vi "Configure DMM.vi"(5 "Resolution in Digits":T1(ring)=enum."5 1/2", 7 "Range":dbl=10.0 format="%.2f", 8 "error in (no error)":errorcluster, 9 "Measurement Type":T2(ring), 11 "niDMM in":refnum<class "niDMM.lvclass">) -> (0 "error out":errorcluster, 3 "niDMM out":refnum<class "niDMM.lvclass">)   [LabVIEW 2021, in "niDMM.lvclass"]
doc: "Configures the NI-DMM"
uses:
  niDMM.lvclass
  niDMM.lvclass/niDMM.ctl
  <instrlib>/niDMM/nidmm.llb/niDMM Resolution in Digits.ctl
  <instrlib>/niDMM/nidmm.llb/niDMM Configure Measurement Digits.vi
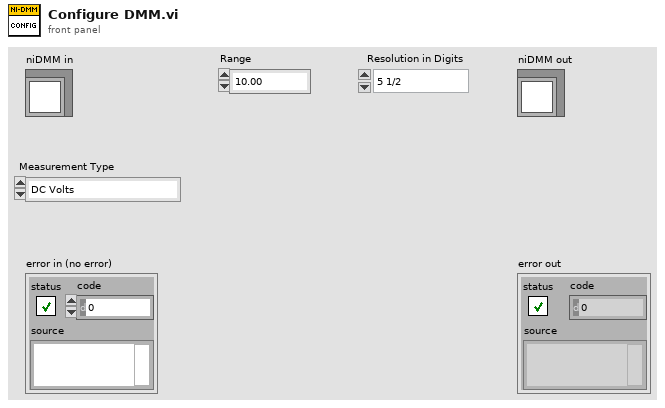
[diagram p1: front panel]
types:
  T1 = enum32{"3 1/2", "4 1/2", "5 1/2", "6 1/2", "7 1/2"}
  T2 = enum32{"DC Volts", "AC Volts", "DC Current", "AC Current", "2-wire Resistance", "4-wire Resistance", "Diode", "Frequency", "Period", "AC Volts DC Coupled", "Capacitance", "Inductance", "Temperature"}
  T3 = typedef "niDMM Resolution in Digits.ctl" = dbl
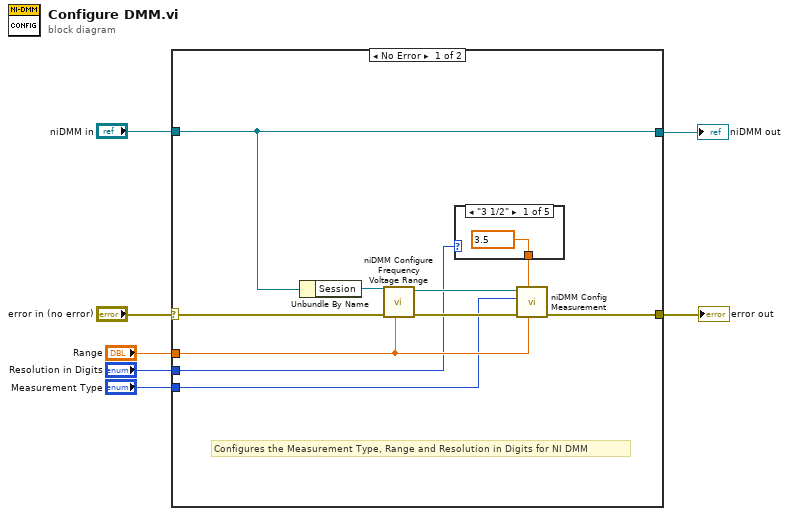
[diagram p0: block diagram]
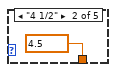
[diagram p2: hidden frame]
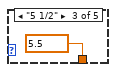
[diagram p3: hidden frame]
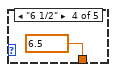
[diagram p4: hidden frame]
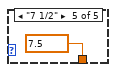
[diagram p5: hidden frame]
diagram:
  n1 = case shown="No Error" "error in (no error)" {
    selector: "error in (no error)" -> [w17 w23]
    tunnel: "niDMM in" -> [w16 w24]
    tunnel: [w16 w24] -> w5
    tunnel: [w15 w23] -> w4
    tunnel: "Range" -> [w10 _]
    tunnel: "Resolution in Digits" -> [w9 _]
    tunnel: "Measurement Type" -> [w8 _]
    frame No Error {
      # "Configures the Measurement Type, Range and Resolution in Digits for NI DMM"
      n2 = Unbundle By Name(w16) -> ("Session"=w11:refnum<k15>)
      n3 = call <instrlib>:"niDMM Configure Frequency Voltage Range.vi"("Frequency Voltage Range"=w10, "error in (no error)"=w17, "instrument handle"=w11) -> ("error out"=w14:errorcluster, "instrument handle out"=w13:refnum<k15>)  [unwired: 7 in]
      n4 = case shown="\"3 1/2\"" w9 {
        tunnel: [w18 w19 w20 w21 w22] -> w12
        frame "3 1/2" {
          w18 = T3 3.5 items=["3 1/2"=3.5, "4 1/2"=4.5, "5 1/2"=5.5, "6 1/2"=6.5, "7 1/2"=7.5] ("Resolution in Digits")
        }
        frame "4 1/2" {
          w19 = T3 4.5 items=["3 1/2"=3.5, "4 1/2"=4.5, "5 1/2"=5.5, "6 1/2"=6.5, "7 1/2"=7.5] ("Resolution in Digits")
        }
        frame "5 1/2" {
          w20 = T3 5.5 items=["3 1/2"=3.5, "4 1/2"=4.5, "5 1/2"=5.5, "6 1/2"=6.5, "7 1/2"=7.5] ("Resolution in Digits")
        }
        frame "6 1/2" {
          w21 = T3 6.5 items=["3 1/2"=3.5, "4 1/2"=4.5, "5 1/2"=5.5, "6 1/2"=6.5, "7 1/2"=7.5] ("Resolution in Digits")
        }
        frame "7 1/2" {
          w22 = T3 7.5 items=["3 1/2"=3.5, "4 1/2"=4.5, "5 1/2"=5.5, "6 1/2"=6.5, "7 1/2"=7.5] ("Resolution in Digits")
        }
      }
      n5 = call-poly <instrlib>:"niDMM Config Measurement.vi"("Range"=w10, "Resolution in Digits"=w12, "error in (no error)"=w14, "Function"=w8, "instrument handle"=w13) -> ("error out"=w15:errorcluster)  [unwired: 5 in, 1 out]
    }
    frame Error {
    }
  }
  "error out" <- w4
  "niDMM out" <- w5
